vi "Destroy Wait Events.vi"(8 "error in (no error)":errorcluster, 11 "Wait User Events":T1) -> (0 "error out":errorcluster)   [LabVIEW 2023, in "Weather Wait Loop.lvlib"]
doc: "Destroys the user events used by the wait message loop."
uses:
  Weather Wait Loop.lvlib
  User Events.ctl
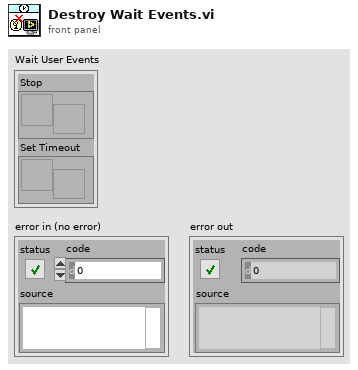
[diagram p1: front panel]
types:
  T1 = typedef "Weather Wait Loop.lvlib/User Events.ctl" = cluster{"Stop":refnum<user-event>, "Set Timeout":refnum<user-event>}
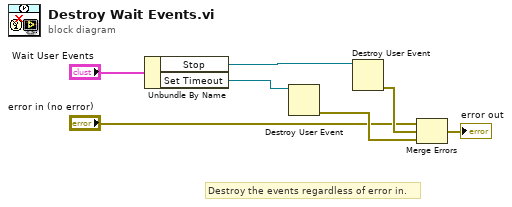
[diagram p0: block diagram]
diagram:
  # "Destroy the events regardless of error in."
  n1 = Unbundle By Name("Wait User Events") -> ("Stop"=w4:refnum<user-event>, "Set Timeout"=w6:refnum<user-event>)
  n2 = Destroy User Event(user event=w6) -> (error out=w2:errorcluster)  [unwired: 1 in]
  n3 = Destroy User Event(user event=w4) -> (error out=w5:errorcluster)  [unwired: 1 in]
  n4 = Merge Errors("error in (no error)", w5, w2) -> (→"error out":errorcluster)
